vi "Read Last Ack Event.vi"(11 "Assert Startup UI in":refnum<class "Assert Startup UI.lvclass">) -> (2 "Last Ack Event":refnum<user-event>)   [LabVIEW 2016, in "Assert Startup UI.lvlib" / "Assert Startup UI.lvclass"]
uses:
  Assert Startup UI.lvclass
  <vilib>/ActorFramework/Message Enqueuer/Message Enqueuer.lvclass
  Assert Startup UI.lvclass/Assert Startup UI.ctl
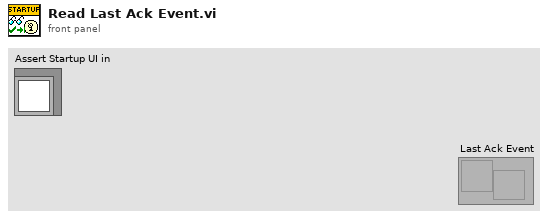
[diagram p1: front panel]
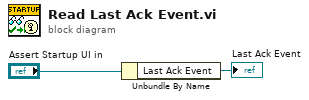
[diagram p0: block diagram]
diagram:
  n1 = Unbundle By Name("Assert Startup UI in") -> ("Last Ack Event"=→"Last Ack Event":refnum<user-event>)
